vi "hasWildcards.vi"(11 "Topic Name (Bytes Array)":u8[](array[numeric])) -> (3 "has Wildcards":bool)   [LabVIEW 2013, in "ControlPacket.lvclass"]
uses:
  ControlPacket.lvclass
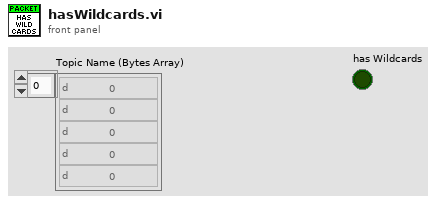
[diagram p1: front panel]
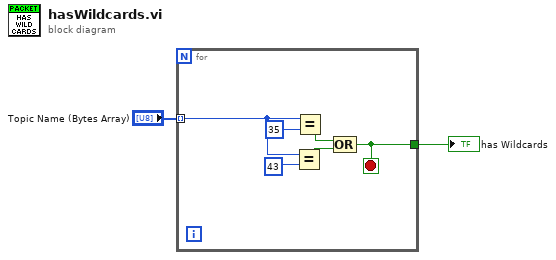
[diagram p0: block diagram]
diagram:
  n1 = for {
    tunnel: "Topic Name (Bytes Array)" -> [w8] mode=indexing
    tunnel: [w5] -> w1
    stop <- w5 stop-if-true
    n2 = Equal?(x=w8, y=u8 43) -> (x = y?=w7:bool)
    n3 = Equal?(x=w8, y=u8 35) -> (x = y?=w6:bool)
    n4 = Compound Arithmetic op=OR(w6, w7) -> (w5:bool)
  }
  "has Wildcards" <- w1
